vi "DSF.Engine.Runtime.Plugin.Get Timing.vi"(8 "error in (no error)":errorcluster, 11 "Plugin Runtime in":refnum<class "DSF.Engine.Runtime.Plugin.lvclass">) -> (0 "error out":errorcluster, 2 "Timing":refnum<class "DSF.Engine.Timing.lvclass">, 3 "Plugin Runtime out":refnum<class "DSF.Engine.Runtime.Plugin.lvclass">)   [LabVIEW 2016, in "DSF.Engine.lvlib" / "DSF.Engine.Runtime.Plugin.lvclass"]
uses:
  DSF.Engine.Runtime.Plugin.lvclass
  Timing/DSF.Engine.Timing.lvclass
  DSF.Engine.Runtime.Plugin.lvclass/DSF.Engine.Runtime.Plugin.ctl
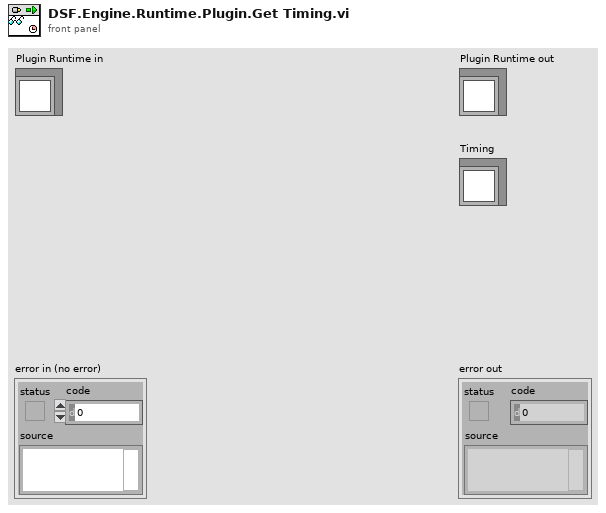
[diagram p1: front panel]
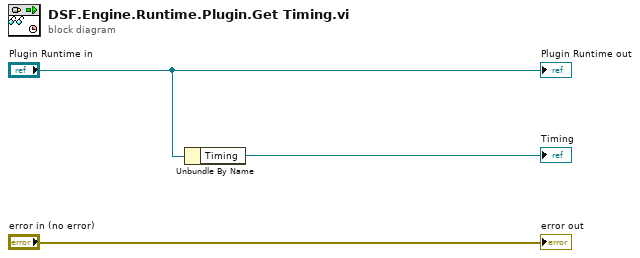
[diagram p0: block diagram]
diagram:
  n1 = Unbundle By Name("Plugin Runtime in") -> ("Timing"=→"Timing":refnum<class "DSF.Engine.Timing.lvclass">)
  "error out" <- "error in (no error)"
  "Plugin Runtime out" <- "Plugin Runtime in"
